vi "PickUpContainer.vi"() -> ()   [LabVIEW 2016, in "LEGO-PMR.lvrbt"]
uses:
  LEGO-PMR.lvrbt
  <vilib>/NXT/Block Support/NXT_OutputPort.ctl
  <vilib>/NXT/NXTIO Xnodes/NXTIONodeSubVIs/NXTMotorRunDistance.vi
  <vilib>/NXT/NXTIO Xnodes/AddressXNode/NXTIOAddress.xnode
  <vilib>/NXT/Subs/LVHSConnector.ctl
  <vilib>/NXT/NXTIO Xnodes/NXTIOXNode/NXTIO.xnode
  <vilib>/NXT/LegoClasses/BrickReference/BrickReference.lvclass
panel:
  out "Up":bool
  in  "Boolean":bool
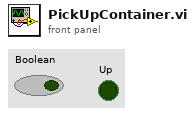
[diagram p1: front panel]
types:
  T1 = typedef "NXT_OutputPort.ctl" = u8
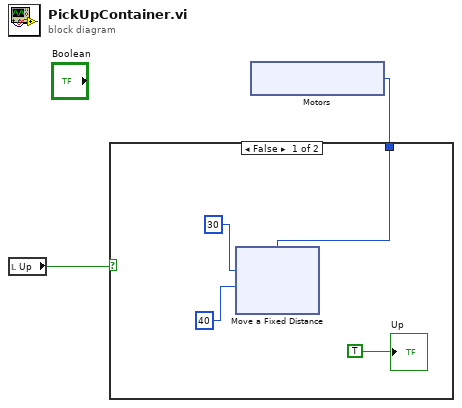
[diagram p0: block diagram]
diagram:
  n1 = local read "Up"() -> (w2:bool)
  n2 = xnode "Motors"() -> ("Motor"=w1:T1)
  n3 = case shown="False" w2 {
    tunnel: w1 -> [w5 _]
    frame False {
      n4 = xnode "Move a Fixed Distance"("Speed 1"=40, "Distance 1"=30, "Motors"=w5) -> ()  [unwired: 1 in, 1 out]
      "Up" <- TRUE
    }
    frame True {
    }
  }
